vi "GetExtensionInfo.vi"(8 "error in (no error)":errorcluster, 11 "FileFormat in":refnum<class "FileFormat.lvclass">) -> (0 "error out":errorcluster, 2 "Extension Info":T1, 3 "FileFormat out":refnum<class "FileFormat.lvclass">)   [LabVIEW 2015, in "File Formats.lvlib" / "FileFormat.lvclass"]
uses:
  FileFormat.lvclass
  Extension Info.ctl
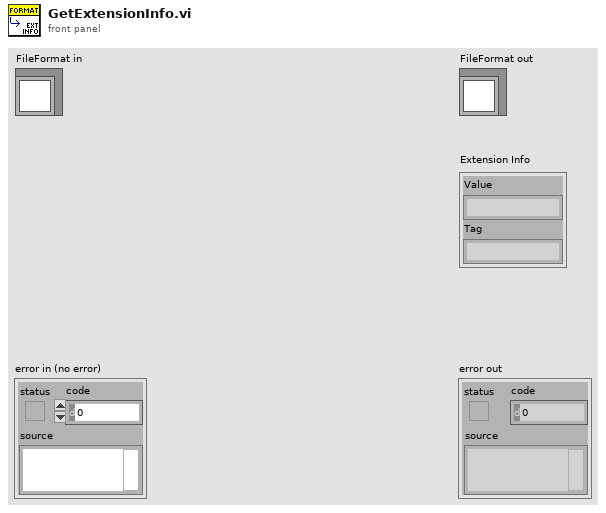
[diagram p1: front panel]
types:
  T1 = typedef "File Formats.lvlib/FileFormat.lvclass/Extension Info.ctl" = cluster{"Value":string, "Tag":string}
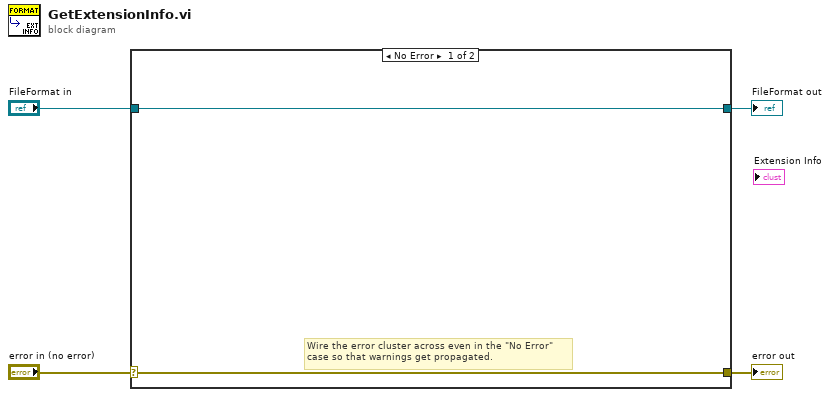
[diagram p0: block diagram]
diagram:
  n1 = case shown="No Error" "error in (no error)" {
    selector: "error in (no error)" -> [w5 w8]
    tunnel: [w5 w8] -> w3
    tunnel: [w6 w7] -> w1
    tunnel: "FileFormat in" -> [w6 w7]
    frame No Error {
      # "Wire the error cluster across even in the \"No Error\"\ncase so that warnings get propagated."
    }
    frame Error {
    }
  }
  "error out" <- w3
  "FileFormat out" <- w1
